vi "Start.vi"() -> ()   [LabVIEW 2015]
panel:
  in  "y 3":dbl
  in  "x 2":dbl
  out "x*y 2":dbl
  out "x*y":dbl
  in  "x":dbl
  in  "y 2":dbl
  out "x+y":dbl
  in  "y":dbl
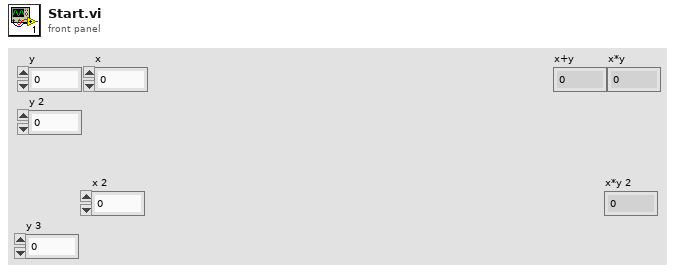
[diagram p1: front panel]
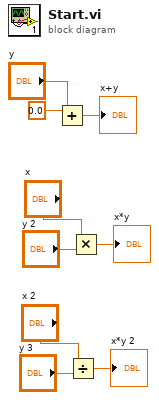
[diagram p0: block diagram]
diagram:
  n1 = Add(x=0.0, y="y") -> (x+y=→"x+y":dbl)
  n2 = Divide(x="x 2", y="y 3") -> (x/y=→"x*y 2":dbl)
  n3 = Multiply(x="x", y="y 2") -> (x*y=→"x*y":dbl)
